vi "Lift Encoder get.vi"(8 "BottomSwitchRef 2":T1={"DevStatus"={"status"=FALSE, "code"=0, "source"=""}, "DIO Channel"=enum."DIO 1", "Controller"=enum."Controller 1"}, 9 "AIDeviceRefLeft":T4={"DevStatus"={"status"=FALSE, "code"=0, "source"=""}, "Controller"=enum."Controller 1", "Analog Channel"=enum."AI 1"}, 10 "BottomSwitchRef":T1={"DevStatus"={"status"=FALSE, "code"=0, "source"=""}, "DIO Channel"=enum."DIO 1", "Controller"=enum."Controller 1"}, 11 "AIDeviceRefRight":T4={"DevStatus"={"status"=FALSE, "code"=0, "source"=""}, "Controller"=enum."Controller 1", "Analog Channel"=enum."AI 1"}) -> ()   [LabVIEW 2014]
uses:
  <vilib>/Rock Robotics/WPI/AnalogChannel/WPI_AnalogChannelDevRef.ctl
  <vilib>/Rock Robotics/SystemInterfaces/Typedef/FPGA_TypedefAnalogModule.ctl
  <vilib>/Rock Robotics/SystemInterfaces/AI/FPGA_AIChannel.ctl
  <vilib>/Rock Robotics/WPI/DigitalInput/WPI_DigitalInputDevRef.ctl
  <vilib>/Rock Robotics/SystemInterfaces/DIO/FPGA_DIOChannel.ctl
  <vilib>/Rock Robotics/SystemInterfaces/Typedef/FPGA_TypedefDigitalModule.ctl
  Robot Values.vi
panel:
  in  "Reset Encoder":bool
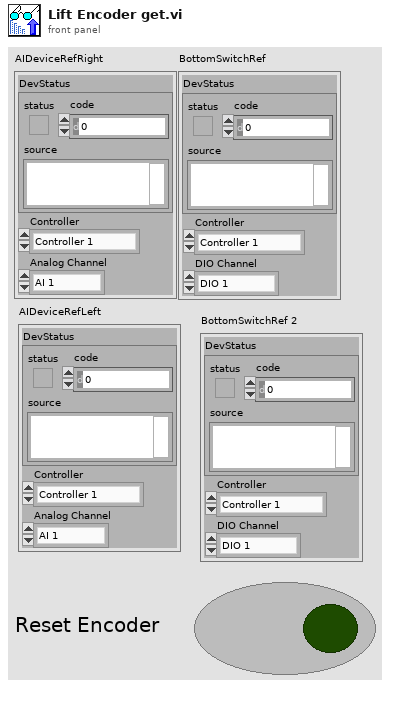
[diagram p1: front panel]
types:
  T1 = typedef "WPI_DigitalInputDevRef.ctl" = cluster{"DevStatus":errorcluster, "DIO Channel":T2, "Controller":T3}
  T2 = typedef "FPGA_DIOChannel.ctl" = enum8{"DIO 0", "DIO 1", "DIO 2", "DIO 3", "DIO 4", "DIO 5", "DIO 6", "DIO 7", "DIO 8", "DIO 9", "DIO MXP 0", "DIO MXP 1", "DIO MXP 2", "DIO MXP 3", "DIO MXP 4", "DIO MXP 5", "DIO MXP 6", "DIO MXP 7", "DIO MXP 8", "DIO MXP 9", "DIO MXP 10", "DIO MXP 11", "DIO MXP 12", "DIO MXP 13", "DIO MXP 14", "DIO MXP 15", "Invalid"}
  T3 = typedef "FPGA_TypedefDigitalModule.ctl" = enum16{"Controller 1"}
  T4 = typedef "WPI_AnalogChannelDevRef.ctl" = cluster{"DevStatus":errorcluster, "Controller":T5, "Analog Channel":T6}
  T5 = typedef "FPGA_TypedefAnalogModule.ctl" = enum16{"Controller 1"}
  T6 = typedef "FPGA_AIChannel.ctl" = enum8{"AI 0", "AI 1", "AI 2", "AI 3", "AI MXP 0", "AI MXP 1", "AI MXP 2", "AI MXP 3", "Invalid"}
  T7 = cluster{"Lift Encoder Height Right (cm)":dbl, "Lift Encoder Height Left (cm)":dbl, "Right Prox":bool, "Left Prox":bool}
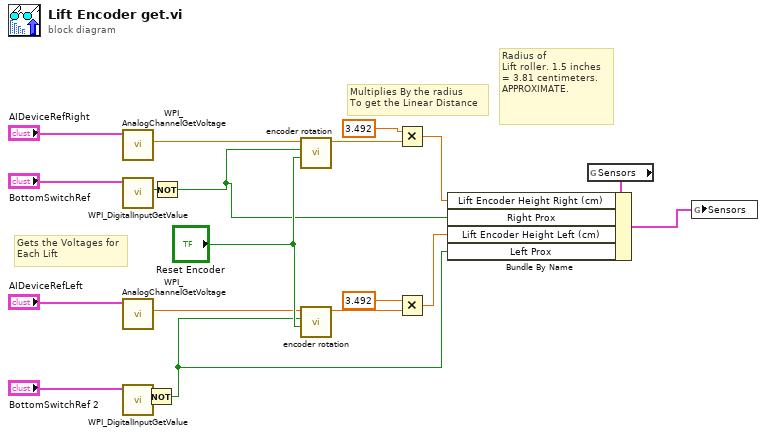
[diagram p0: block diagram]
diagram:
  # "Multiplies By the radius\nTo get the Linear Distance"
  # "Gets the Voltages for\nEach Lift"
  # "Radius of\nLift roller. 1.5 inches = 3.81 centimeters. APPROXIMATE."
  n1 = call <vilib>:"WPI_AnalogChannelGetVoltage.vi"("AIDeviceRef"="AIDeviceRefRight") -> ("Voltage"=w5:dbl)  [unwired: 8 in, 2 out]
  n2 = call <vilib>:"WPI_DigitalInputGetValue.vi"("DigitalInputDevRef"="BottomSwitchRef") -> ("Value"=w4:bool)  [unwired: 8 in, 2 out]
  n3 = call <vilib>:"WPI_AnalogChannelGetVoltage.vi"("AIDeviceRef"="AIDeviceRefLeft") -> ("Voltage"=w7:dbl)  [unwired: 8 in, 2 out]
  n4 = call <vilib>:"WPI_DigitalInputGetValue.vi"("DigitalInputDevRef"="BottomSwitchRef 2") -> ("Value"=w10:bool)  [unwired: 8 in, 2 out]
  n5 = Not(x=w10) -> (.not. x?=w1:bool)
  n6 = Not(x=w4) -> (.not. x?=w2:bool)
  n7 = call "encoder rotation.vi"("Reset Encoder"="Reset Encoder", "Switch value"=w2, "Voltage"=w5) -> ("Angle(rad)"=w13:dbl)  [unwired: 6 in, 2 out]
  n8 = call "encoder rotation.vi"("Reset Encoder"="Reset Encoder", "Switch value"=w1, "Voltage"=w7) -> ("Angle(rad)"=w12:dbl)  [unwired: 6 in, 2 out]
  n9 = Multiply(x=3.492, y=w13) -> (x*y=w16:dbl)
  n10 = Multiply(x=3.492, y=w12) -> (x*y=w14:dbl)
  n11 = global read "Robot Values.vi" "Sensors"() -> (w18:T7)
  n12 = Bundle By Name(cluster=w18, "Lift Encoder Height Right (cm)"=w16, "Right Prox"=w2, "Lift Encoder Height Left (cm)"=w14, "Left Prox"=w1) -> (w19:T7)
  n13 = global write "Robot Values.vi" "Sensors"(w19) -> ()
